vi "Configure Acquisition.vi"(8 "error in":errorcluster, 11 "Continuous Waveform Acq CFG in":refnum<class "Continuous Waveform Acq CFG.lvclass">) -> (0 "error out":errorcluster, 3 "Continuous Waveform Acq CFG out":refnum<class "Continuous Waveform Acq CFG.lvclass">)   [LabVIEW 2023, in "Continuous Waveform Acq CFG.lvclass"]
uses:
  Continuous Waveform Acq CFG.lvclass
  Continuous Waveform Acq CFG.lvclass/Continuous Waveform Acq CFG.ctl
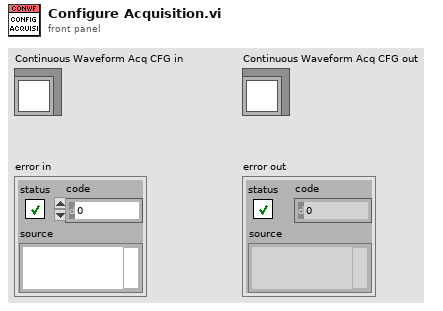
[diagram p1: front panel]
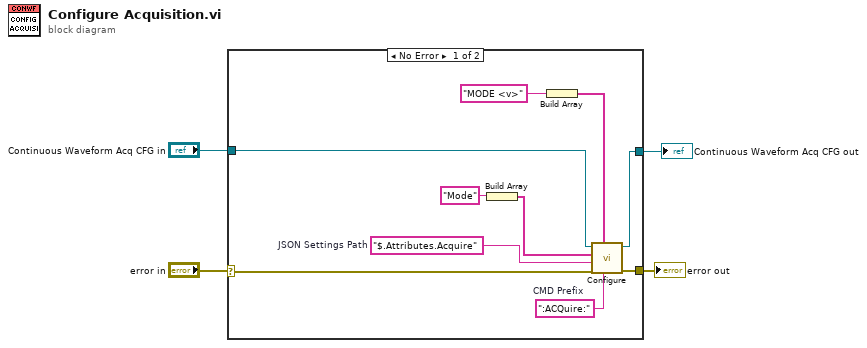
[diagram p0: block diagram]
diagram:
  n1 = case shown="No Error" "error in" {
    selector: "error in" -> [w6 w16]
    tunnel: [w14 w16] -> w4
    tunnel: [w13 w15] -> w3
    tunnel: "Continuous Waveform Acq CFG in" -> [w5 w15]
    frame No Error {
      w12 = ":ACQuire:"  # CMD Prefix
      w11 = "$.Attributes.Acquire"  # JSON Settings Path
      n2 = Build Array("Mode") -> (w7:string[])
      n3 = Build Array("MODE <v>") -> (w9:string[])
      n4 = call "Configure.vi"("CMD Prefix"=w12, "CMDs"=w9, "error in"=w6, "JSON Settings Path"=w11, "JSON Keys"=w7, "Continuous Waveform Acq CFG in"=w5) -> ("error out"=w14:errorcluster, "Continuous Waveform Acq CFG out"=w13:refnum<class "Continuous Waveform Acq CFG.lvclass">)  [unwired: 4 in]
    }
    frame Error {
    }
  }
  "error out" <- w4
  "Continuous Waveform Acq CFG out" <- w3
